vi "scan_waveformTriangle_fred.vi"(5 "y flyback":bool, 6 "nlines":i32, 7 "y flyback":dbl, 8 "flyback":i32, 9 "xpixels":i32, 10 "maxV":dbl, 11 "minV":dbl) -> (2 "xy scan waveform":dbl[][](array[numeric]))   [LabVIEW 2010]
panel:
  out "size(s) 2":i32
  out "size(s)":i32
  out "x waveform":dbl[](graph)
  out "y waveform":dbl[](graph)
  out "ystepSize":dbl
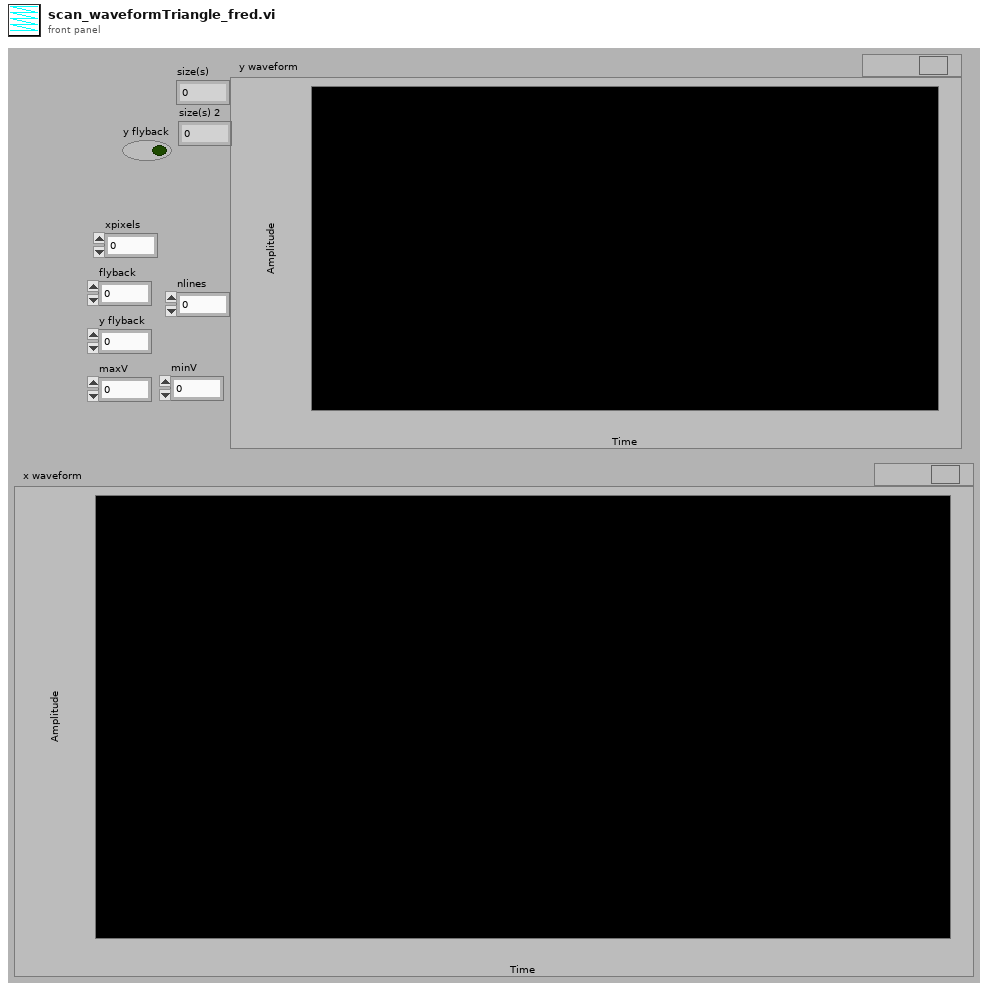
[diagram p1: front panel]
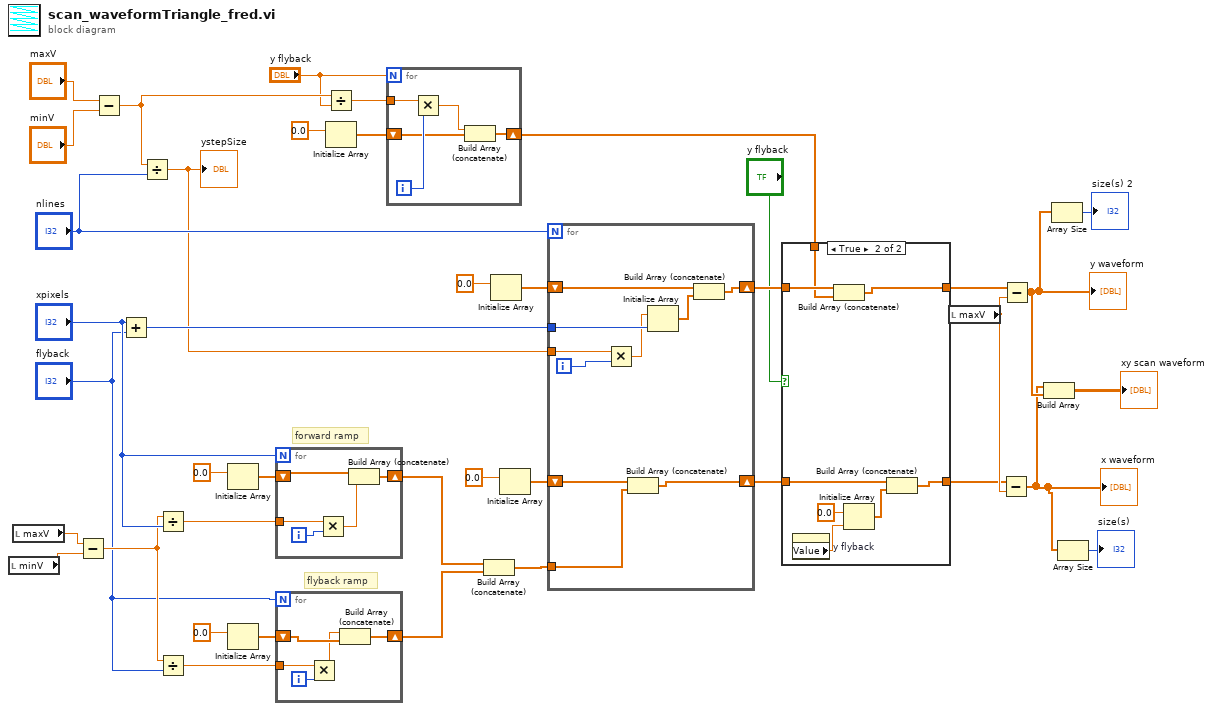
[diagram p0: block diagram]
diagram:
  # "flyback ramp"
  # "forward ramp"
  n1 = local read "minV"() -> (w31:dbl)
  n2 = local read "maxV"() -> (w32:dbl)
  n3 = Subtract(x=w32, y=w31) -> (x-y=w20:dbl)
  n4 = Subtract(x="maxV", y="minV") -> (x-y=w7:dbl)
  n5 = Add(x="xpixels", y="flyback") -> (x+y=w35:i32)
  n6 = Divide(x=w7, y="nlines") -> (x/y=w17:dbl)
  "ystepSize" <- w17
  n7 = Divide(x=w20, y="xpixels") -> (x/y=w28:dbl)
  n8 = Divide(x=w20, y="flyback") -> (x/y=w27:dbl)
  n9 = Initialize Array(0.0 ("element")) -> (w33:dbl[])  [unwired: 1 out]
  n10 = Initialize Array(0.0 ("element")) -> (w30:dbl[])  [unwired: 1 out]
  n11 = for {
    N: "xpixels" -> [_]
    tunnel: w28 -> [w43]
    shift-right: [w41] -> w26
    shift-left: w33 -> [w45]
    i -> [w44]
    n12 = Multiply(x=w43, y=w44) -> (x*y=w42:dbl)
    n13 = Build Array (concatenate)(w45, w42) -> (w41:dbl[])
  }
  n14 = for {
    N: "flyback" -> [_]
    tunnel: w27 -> [w50]
    shift-right: [w48] -> w18
    shift-left: w30 -> [w47]
    i -> [w49]
    n15 = Multiply(x=w50, y=w49) -> (x*y=w46:dbl)
    n16 = Build Array (concatenate)(w46, w47) -> (w48:dbl[])
  }
  n17 = Divide(x=w7, y="y flyback") -> (x/y=w14:dbl)
  n18 = Initialize Array(0.0 ("element")) -> (w15:dbl[])  [unwired: 1 out]
  n19 = for {
    N: "y flyback" -> [_]
    shift-right: [w51] -> w8
    shift-left: w15 -> [w52]
    tunnel: w14 -> [w55]
    i -> [w54]
    n20 = Multiply(x=w55, y=w54) -> (x*y=w53:dbl)
    n21 = Build Array (concatenate)(w53, w52) -> (w51:dbl[])
  }
  n22 = Build Array (concatenate)(w26, w18) -> (w23:dbl[])
  n23 = Initialize Array(0.0 ("element")) -> (w40:dbl[])  [unwired: 1 out]
  n24 = Initialize Array(0.0 ("element")) -> (w24:dbl[])  [unwired: 1 out]
  n25 = for {
    N: "nlines" -> [_]
    tunnel: w17 -> [w63]
    tunnel: w35 -> [w65]
    shift-right: [w59] -> w12
    shift-left: w40 -> [w60]
    shift-right: [w56] -> w13
    shift-left: w24 -> [w57]
    tunnel: w23 -> [w58]
    i -> [w64]
    n26 = Multiply(x=w63, y=w64) -> (x*y=w62:dbl)
    n27 = Build Array (concatenate)(w57, w58) -> (w56:dbl[])
    n28 = Initialize Array(w62, w65) -> (w61:dbl[])
    n29 = Build Array (concatenate)(w60, w61) -> (w59:dbl[])
  }
  n30 = case shown="True" "y flyback" {
    tunnel: w13 -> [w66 w70]
    tunnel: w12 -> [w67 w75]
    tunnel: [w67 w73] -> w9
    tunnel: [w66 w72] -> w10
    tunnel: w8 -> [_ w74]
    frame False {
    }
    frame True {
      n31 = property on="y flyback" class="DigNum (strict)"() -> ("Value"=w69:dbl)  [unwired: 2 in, 2 out]
      n32 = Build Array (concatenate)(w75, w74) -> (w73:dbl[])
      n33 = Initialize Array(0.0 ("element"), w69) -> (w71:dbl[])
      n34 = Build Array (concatenate)(w70, w71) -> (w72:dbl[])
    }
  }
  n35 = local read "maxV"() -> (w22:dbl)
  n36 = Subtract(x=w10, y=w22) -> (x-y=w4:dbl[])
  "x waveform" <- w4
  n37 = Subtract(x=w9, y=w22) -> (x-y=w5:dbl[])
  "y waveform" <- w5
  n38 = Build Array(w4, w5) -> (→"xy scan waveform":dbl[][])
  n39 = Array Size(array=w5) -> (size(s)=→"size(s) 2":i32)
  n40 = Array Size(array=w4) -> (size(s)=→"size(s)":i32)
